vi "ACR_READ.vi"(8 "error in (no error)":errorcluster, 10 "Actual":string, 11 "Automation Refnum in":refnum<k7>) -> (0 "error out":errorcluster, 3 "AXIS0":dbl)   [LabVIEW 2015]
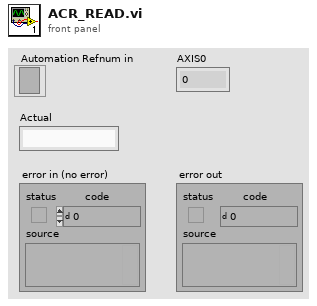
[diagram p1: front panel]
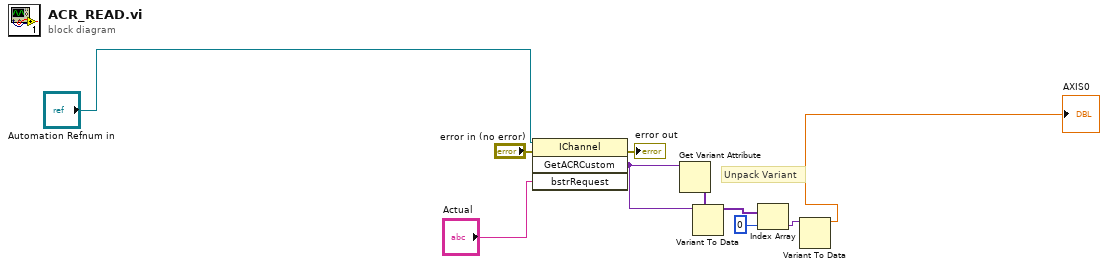
[diagram p0: block diagram]
diagram:
  # "Unpack Variant"
  n1 = invoke class="IChannel" method="GetACRCustom"(reference="Automation Refnum in", error in="error in (no error)", "bstrRequest"="Actual") -> (error out=→"error out":errorcluster, "GetACRCustom"=w4:variant)  [unwired: 1 in, 2 out]
  n2 = Get Variant Attribute(Variant=w4) -> (values=w3:variant[])  [unwired: 1 in, 5 out]
  n3 = Variant To Data(type=w3, Variant=w4) -> (data=w5:variant[])  [unwired: 1 in, 1 out]
  n4 = Index Array(array=w5, index=0) -> (element=w7:variant)
  n5 = Variant To Data(Variant=w7) -> (data=→"AXIS0":dbl)  [unwired: 2 in, 1 out]
